vi "test-path-planner-read-csv.vi"() -> ()   [LabVIEW 2019]
uses:
  <vilib>/Rock Robotics/WPI/ThirdParty/MJansen/PathPlanner/TypeDef/PathPlannerTrajectory.ctl
  <vilib>/Rock Robotics/WPI/ThirdParty/MJansen/PathPlanner/TypeDef/PathPlannerTrajectoryState.ctl
  <vilib>/Rock Robotics/WPI/ThirdParty/JAS_Junk/TrajLib/TypeDef/TRANSLATION2D.ctl
  <vilib>/Rock Robotics/WPI/ThirdParty/JAS_Junk/TrajLib/TypeDef/ROTATION2D.ctl
  <vilib>/Rock Robotics/WPI/ThirdParty/MJansen/PathPlanner/TypeDef/PathPlannerPathConstraints.ctl
  <vilib>/Rock Robotics/WPI/ThirdParty/JAS_Junk/TrajLib/TypeDef/TRAJ_STATE.ctl
  <vilib>/Rock Robotics/WPI/ThirdParty/JAS_Junk/TrajLib/TypeDef/POSE2D.ctl
  <vilib>/Rock Robotics/WPI/ThirdParty/MJansen/PathPlanner/PathPlanner24.lvlib
  <vilib>/Rock Robotics/WPI/ThirdParty/JAS_Junk/TrajLib/Trajectory_Library.lvlib
panel:
  in  "Tab Control":T1(tab)
  in  "stop":bool
  in  "Path FileName":string="C:\\Shares\\github\\PathPlannerLabVIEW\\PathPlannerSandbox24\\PathPlannerTestCSV\\PathPlannerTestCSV.csv"
  out "Full FIlename":string
  out "error out":errorcluster
  out "PathPlannerTrajectory":T2 {"States"."TargetHolonomicRotation"."SIN" format="%13.4f"; "States"."TargetHolonomicRotation"."COS" format="%13.4f"; "States"."TargetHolonomicRotation"."VALUE" format="%13.4f"; "States"."Heading"."SIN" format="%13.4f"; "States"."Heading"."COS" format="%13.4f"; "States"."Heading"."VALUE" format="%13.4f"; "States"."PositionMeters"."Y" format="%14.3f"; "States"."PositionMeters"."X" format="%14.3f"}
  out "outPathPlannerStates":T3[](array[typedef]) {"TargetHolonomicRotation"."SIN" format="%13.4f"; "TargetHolonomicRotation"."COS" format="%13.4f"; "TargetHolonomicRotation"."VALUE" format="%13.4f"; "Heading"."SIN" format="%13.4f"; "Heading"."COS" format="%13.4f"; "Heading"."VALUE" format="%13.4f"; "PositionMeters"."Y" format="%14.3f"; "PositionMeters"."X" format="%14.3f"}
  in  "Down Button":bool
  in  "Up Button":bool
  in  "index":i32 step=20
  out "LabVIEWStateCount":i32
  out "LabVIEWStates":T7[](array[typedef]) {"POSE"."ROTATION"."SIN" format="%13.4f"; "POSE"."ROTATION"."COS" format="%13.4f"; "POSE"."ROTATION"."VALUE" format="%13.4f"; "POSE"."TRANSLATION"."Y" format="%14.3f"; "POSE"."TRANSLATION"."X" format="%14.3f"}
  out "XY SPLINE":cluster{dbl[], dbl[]}[](graph)
  out "XY Graph":cluster{dbl[], dbl[]}[](graph)
  out "Sample Graph":dbl[][](graph)
  out "LabVIEW Time Plot":cluster{dbl[], dbl[]}[](graph)
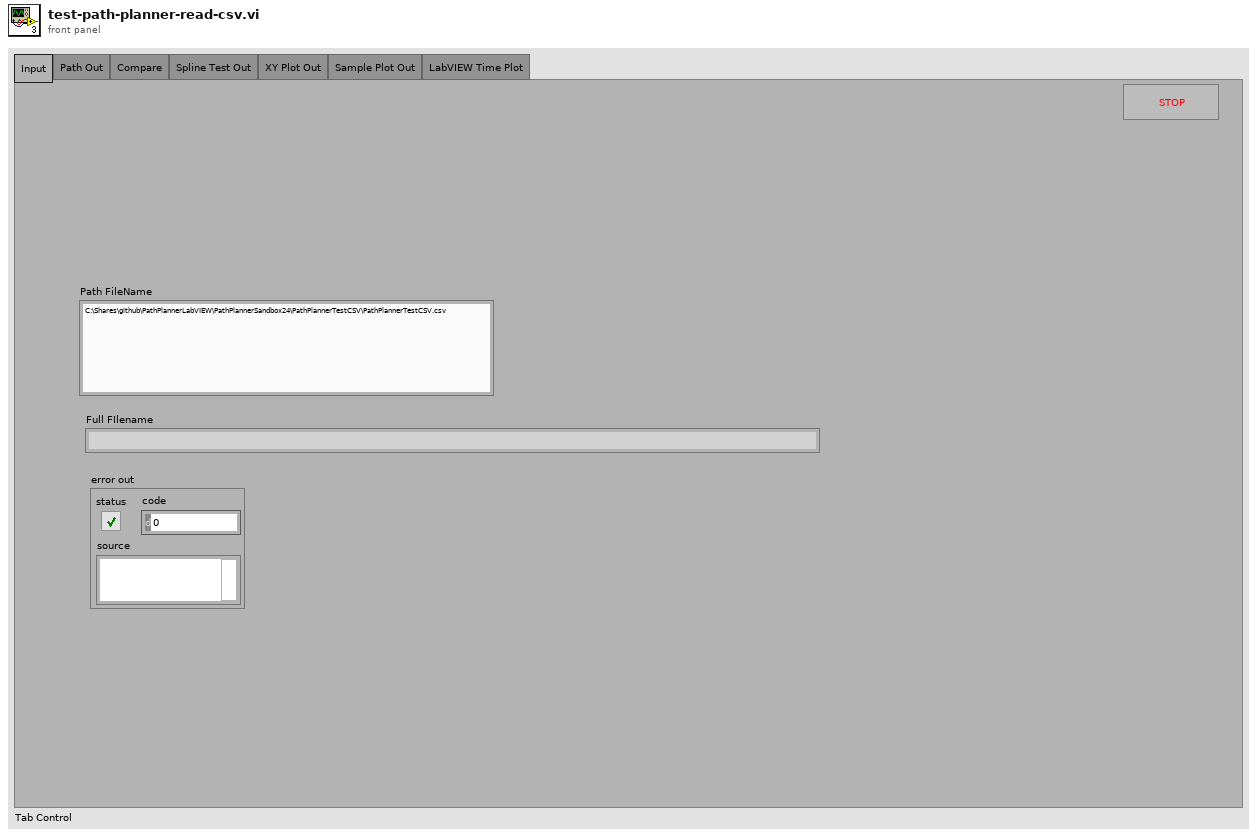
[diagram p1: front panel]
types:
  T1 = enum32{"Input", "Path Out", "Compare", "Spline Test Out", "XY Plot Out", "Sample Plot Out", "LabVIEW Time Plot"}
  T2 = typedef "PathPlanner24.lvlib/PathPlannerTrajectory.ctl" = cluster{"States":T3[]}
  T3 = typedef "PathPlanner24.lvlib/PathPlannerTrajectoryState.ctl" = cluster{"TimeSeconds":dbl, "VelocityMPS":dbl, "AccerationMpsSq":dbl, "HeadingAngularVelRadPerSec":dbl, "PositionMeters":T4, "Heading":T5, "TargetHolonomicRotation":T5, "CurvatureRadPerMeter":dbl, "DeltaPos":dbl, "PathPlannerConstraints":T6}
  T4 = typedef "Trajectory_Library.lvlib/TRANSLATION2D.ctl" = cluster{"X":dbl, "Y":dbl}
  T5 = typedef "Trajectory_Library.lvlib/ROTATION2D.ctl" = cluster{"VALUE":dbl, "COS":dbl, "SIN":dbl}
  T6 = typedef "PathPlanner24.lvlib/PathPlannerPathConstraints.ctl" = cluster{"MaxVelocityMps;":dbl, "MaxAccelerationMpsSq;":dbl, "MaxAngularVelRadPsEc;":dbl, "MaxAngularAccRadPSecSq":dbl, "Exists":bool}
  T7 = typedef "Trajectory_Library.lvlib/TRAJ_STATE.ctl" = cluster{"TimeSeconds":dbl, "Velocity":dbl, "Acceleration":dbl, "POSE":T8, "Curvature":dbl}
  T8 = typedef "Trajectory_Library.lvlib/POSE2D.ctl" = cluster{"TRANSLATION":T4, "ROTATION":T5}
  T9 = typedef "Trajectory_Library.lvlib/TRAJECTORY.ctl" = cluster{"TotalTImeSecs":dbl, "States":T7[]}
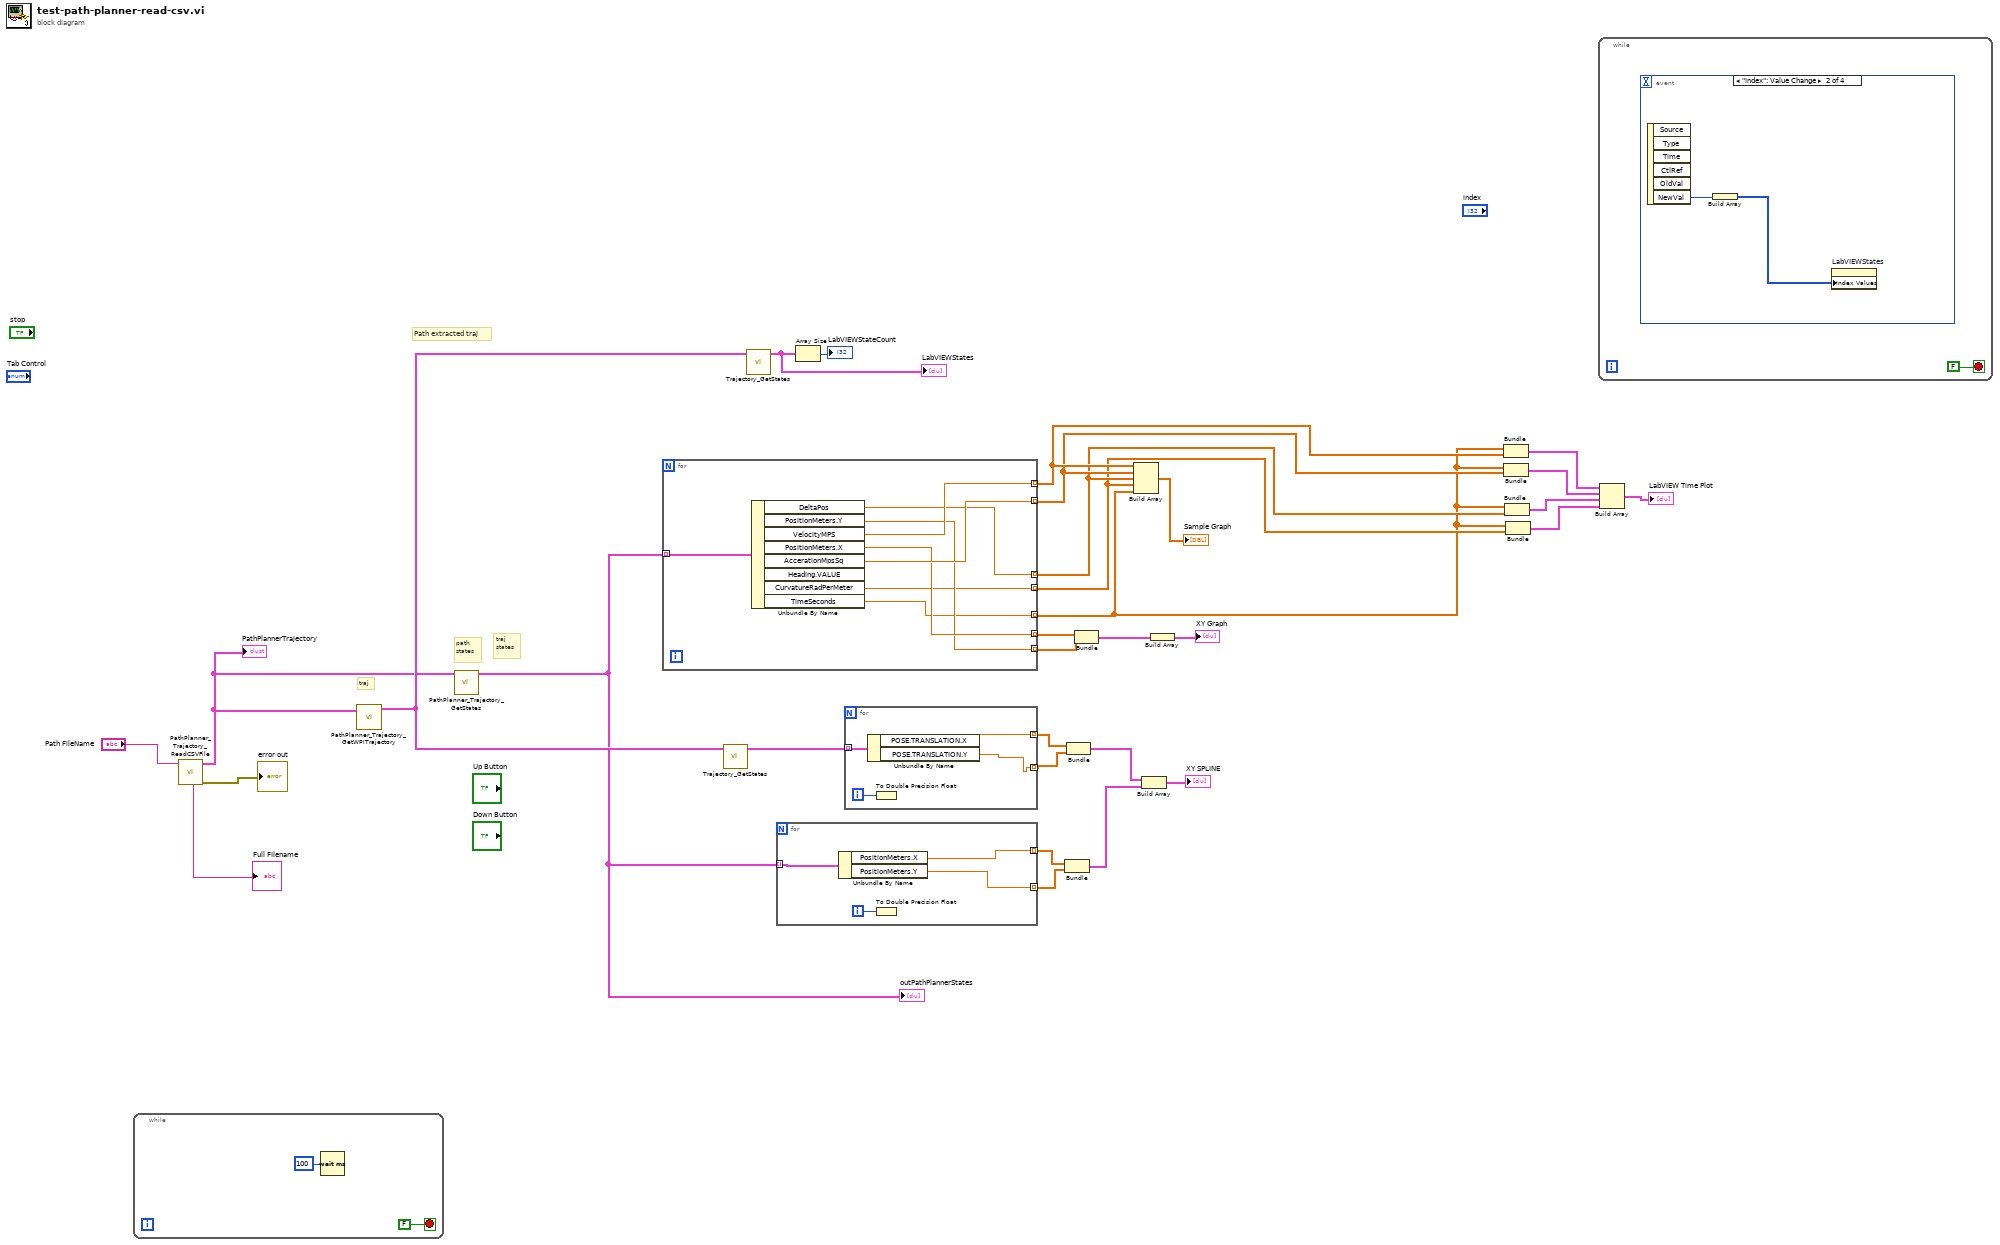
[diagram p0: block diagram]
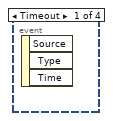
[diagram p2: hidden frame]
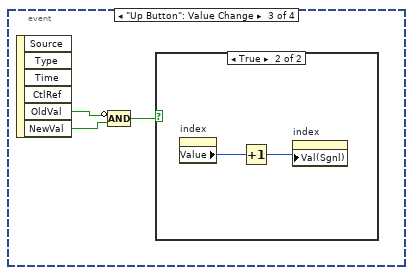
[diagram p3: hidden frame]
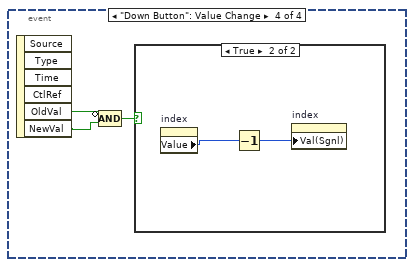
[diagram p5: hidden frame]
diagram:
  # "Path extracted traj"
  # "traj"
  # "traj\nstates"
  # "path\nstates"
  n1 = while {
    stop <- FALSE stop-if-true
    n2 = Wait (ms)(milliseconds to wait=u32 100) -> ()  [unwired: 1 out]
  }
  n3 = call <vilib>:"PathPlanner_Trajectory_ReadCSVFile.vi"("FileName"="Path FileName") -> ("error out"=→"error out":errorcluster, "outTRAJECTORY"=w2:T2, "Full FIlename"=→"Full FIlename":string)  [unwired: 8 in]
  "PathPlannerTrajectory" <- w2
  n4 = call <vilib>:"PathPlanner_Trajectory_GetWPITrajectory.vi"("PathPlannerTrajectory"=w2) -> ("TRAJECTORY"=w18:T9)  [unwired: 9 in, 1 out]
  n5 = call <vilib>:"PathPlanner_Trajectory_GetStates.vi"("PathPlannerTrajectory"=w2) -> ("PathPlannerStates"=w15:T3[])  [unwired: 10 in]
  "outPathPlannerStates" <- w15
  n6 = for {
    tunnel: [w41] -> w13 mode=indexing
    tunnel: [w40] -> w12 mode=indexing
    tunnel: [w35] -> w11 mode=indexing
    tunnel: [w39] -> w30 mode=indexing
    tunnel: [w38] -> w29 mode=indexing
    tunnel: w15 -> [w37] mode=indexing
    tunnel: [w36] -> w10 mode=indexing
    tunnel: [w34] -> w1 mode=indexing
    n7 = Unbundle By Name(w37) -> ("DeltaPos"=w35:dbl, "PositionMeters.Y"=w38:dbl, "VelocityMPS"=w41:dbl, "PositionMeters.X"=w39:dbl, "AccerationMpsSq"=w40:dbl, "CurvatureRadPerMeter"=w36:dbl, "TimeSeconds"=w34:dbl)  [unwired: 1 out]
  }
  n8 = call <vilib>:"Trajectory_GetStates.vi"("TRAJECTORY"=w18) -> ("States"=w19:T7[])  [unwired: 10 in]
  n9 = call <vilib>:"Trajectory_GetStates.vi"("TRAJECTORY"=w18) -> ("States"=w16:T7[])  [unwired: 10 in]
  "LabVIEWStates" <- w16
  n10 = for {
    tunnel: [w44] -> w24 mode=indexing
    tunnel: w15 -> [w43] mode=indexing
    tunnel: [w42] -> w23 mode=indexing
    i -> [w45]
    n11 = Unbundle By Name(w43) -> ("PositionMeters.X"=w44:dbl, "PositionMeters.Y"=w42:dbl)
    n12 = To Double Precision Float(number=w45) -> ()  [unwired: 1 out]
  }
  n13 = Array Size(array=w16) -> (size(s)=→"LabVIEWStateCount":i32)
  n14 = for {
    tunnel: [w48] -> w26 mode=indexing
    tunnel: [w47] -> w25 mode=indexing
    tunnel: w19 -> [w46] mode=indexing
    i -> [w49]
    n15 = Unbundle By Name(w46) -> ("POSE.TRANSLATION.X"=w48:dbl, "POSE.TRANSLATION.Y"=w47:dbl)
    n16 = To Double Precision Float(number=w49) -> ()  [unwired: 1 out]
  }
  n17 = Bundle(w24, w23) -> (w21:cluster{dbl[], dbl[]})  [unwired: 1 in]
  n18 = Bundle(w26, w25) -> (w22:cluster{dbl[], dbl[]})  [unwired: 1 in]
  n19 = Bundle(w30, w29) -> (w28:cluster{dbl[], dbl[]})  [unwired: 1 in]
  n20 = Build Array(w13, w12, w11, w10, w1) -> (→"Sample Graph":dbl[][])
  n21 = Build Array(w22, w21) -> (→"XY SPLINE":cluster{dbl[], dbl[]}[])
  n22 = Build Array(w28) -> (→"XY Graph":cluster{dbl[], dbl[]}[])
  n23 = Bundle(w1, w13) -> (w9:cluster{dbl[], dbl[]})  [unwired: 1 in]
  n24 = Bundle(w1, w12) -> (w8:cluster{dbl[], dbl[]})  [unwired: 1 in]
  n25 = Bundle(w1, w11) -> (w7:cluster{dbl[], dbl[]})  [unwired: 1 in]
  n26 = Bundle(w1, w10) -> (w6:cluster{dbl[], dbl[]})  [unwired: 1 in]
  n27 = while {
    stop <- FALSE stop-if-true
    n28 = event shown="[1] \"index\": Value Change" {
      selector: _ -> [_ _ _ _]
      dyn-events: _ -> [_ _ _ _]
      timeout: _ -> [_ _ _ _]
      event Timeout {
        n29 = event-data() -> ()  [unwired: 1 in, 3 out]
      }
      event "index": Value Change {
        n30 = event-data() -> ("NewVal"=w52:i32)  [unwired: 1 in, 5 out]
        n31 = Build Array(w52) -> (w51:i32[])
        n32 = property on="LabVIEWStates" class="Arr (strict)"("Index Values"=w51) -> ()  [unwired: 2 in, 2 out]
      }
      event "Up Button": Value Change {
        n33 = event-data() -> ("OldVal"=w55:bool, "NewVal"=w54:bool)  [unwired: 1 in, 4 out]
        n34 = Compound Arithmetic op=AND(invert w55, w54) -> (w53:bool)
        n35 = case shown="True" w53 {
          frame False {
          }
          frame True {
            n36 = property on="index" class="DigNum (strict)"() -> ("Value"=w56:i32)  [unwired: 2 in, 2 out]
            n37 = Increment(x=w56) -> (x+1=w57:i32)
            n38 = property on="index" class="DigNum (strict)"("Val(Sgnl)"=w57) -> ()  [unwired: 2 in, 2 out]
          }
        }
      }
      event "Down Button": Value Change {
        n39 = event-data() -> ("OldVal"=w59:bool, "NewVal"=w58:bool)  [unwired: 1 in, 4 out]
        n40 = Compound Arithmetic op=AND(invert w59, w58) -> (w60:bool)
        n41 = case shown="True" w60 {
          frame False {
          }
          frame True {
            n42 = property on="index" class="DigNum (strict)"() -> ("Value"=w61:i32)  [unwired: 2 in, 2 out]
            n43 = Decrement(x=w61) -> (x-1=w62:i32)
            n44 = property on="index" class="DigNum (strict)"("Val(Sgnl)"=w62) -> ()  [unwired: 2 in, 2 out]
          }
        }
      }
    }
  }
  n45 = Build Array(w9, w8, w7, w6) -> (→"LabVIEW Time Plot":cluster{dbl[], dbl[]}[])
